vi "Coaxial RF generator control.vi"() -> ()   [LabVIEW 2021]
uses:
  <vilib>/LabVIEW Interface for Arduino/Type Defs/Pin Mode.ctl
  <vilib>/LabVIEW Interface for Arduino/LabVIEW Interface for Arduino.lvlib
panel:
  in  "Generator on/off":bool
  out "Plasma OFF":bool
  out "NOT signal":bool
  out "Plasma ON":bool
  in  "Enable RF On":bool
  in  "Set power / %":dbl min=0.0 max=100.0 step=0.2
  in  "Turn plasma On":bool
  in  "Enable Set Power":bool
  out "Fwd power":dbl format="%#.1g"
  out "Ref power":dbl format="%#.1g"
  out "Ref power":dbl(knob) scale=0.0..15.0
  out "Fwd power":u32(knob) scale=0.0..150.0
  out "error out":errorcluster
  in  "Stopp":bool
  # "Plasma"
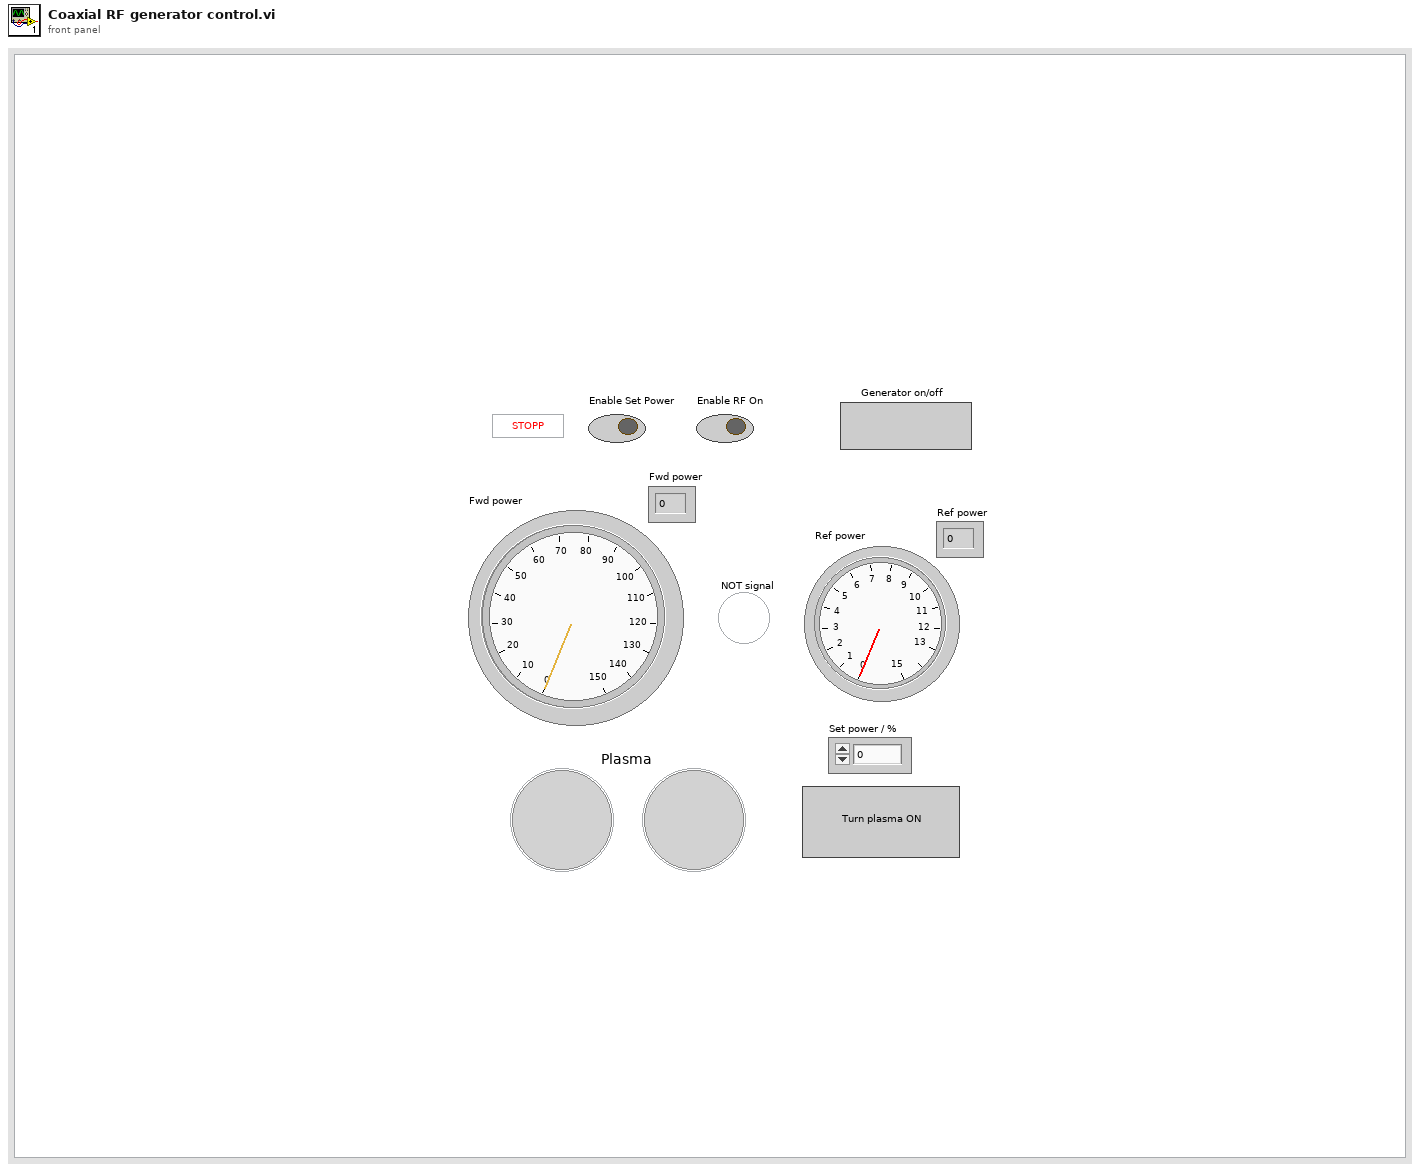
[diagram p1: front panel]
types:
  T1 = typedef "LabVIEW Interface for Arduino.lvlib/Pin Mode.ctl" = enum8{"Input", "Output"}
  T2 = typedef "LabVIEW Interface for Arduino.lvlib/Arduino Resource.ctl" = cluster{"VISA resource":refnum<visa-resource-name>, "Board Type":T3, "Connection Type":enum8{"USB / Serial"}, "Bytes Per Packet (15)":u8}
  T3 = typedef "LabVIEW Interface for Arduino.lvlib/Board Type.ctl" = enum16{"Uno", "Dimuelanove w/Atmega 328", "Mega 2560"}
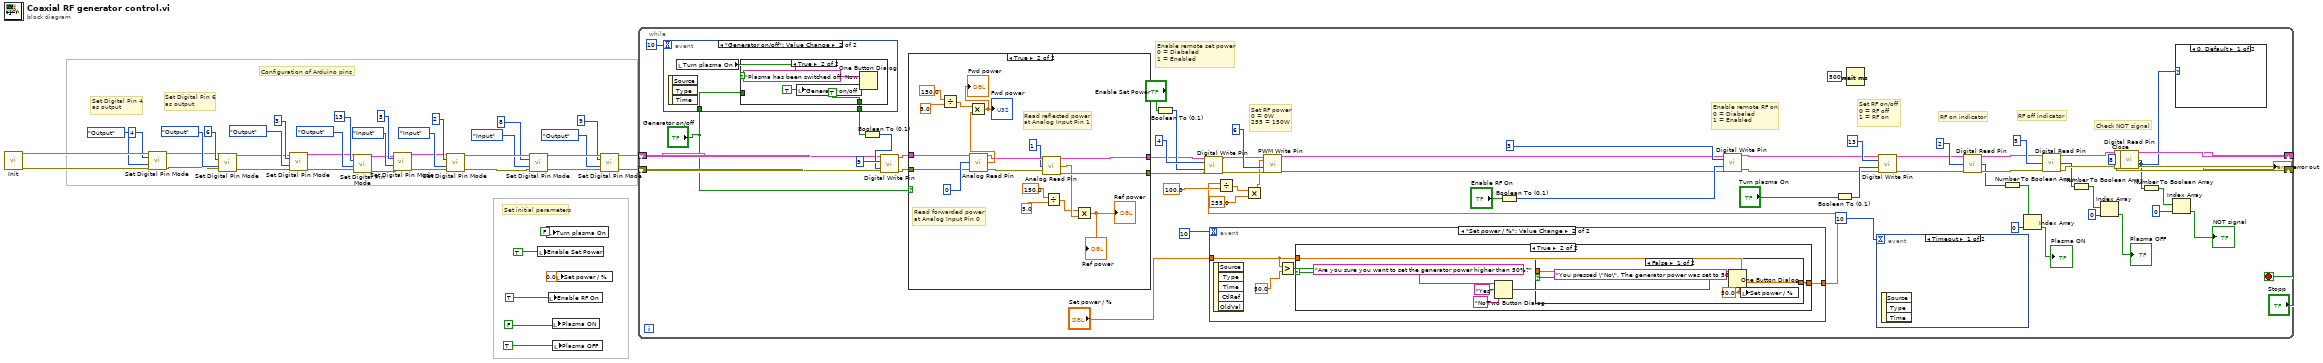
[diagram p0: block diagram]
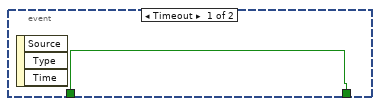
[diagram p2: hidden frame]
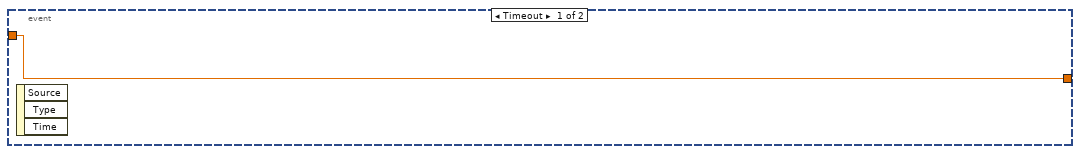
[diagram p4: hidden frame]
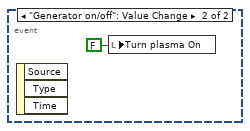
[diagram p8: hidden frame]
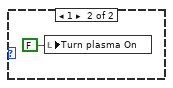
[diagram p9: hidden frame]
diagram:
  # "Configuration of Arduino pins"
  # "Set initial parameters"
  # "Set Digital Pin 6 \nas output"
  # "Set Digital Pin 4 \nas output"
  n1 = call <vilib>:"Init.vi"() -> ("Arduino Resource"=w38:T2, "error out"=w37:errorcluster)  [unwired: 18 in]
  n2 = call <vilib>:"Set Digital Pin Mode.vi"("Arduino Resource"=w38, "Digital I/O Pin"=u8 4, "Pin Mode (Input)"=Pin_Mode."Output", "error in"=w37) -> ("Arduino Resource"=w34:T2, "error out"=w33:errorcluster)  [unwired: 10 in]
  n3 = call <vilib>:"Set Digital Pin Mode.vi"("Arduino Resource"=w34, "Digital I/O Pin"=u8 6, "Pin Mode (Input)"=Pin_Mode."Output", "error in"=w33) -> ("Arduino Resource"=w26:T2, "error out"=w25:errorcluster)  [unwired: 10 in]
  n4 = call <vilib>:"Set Digital Pin Mode.vi"("Arduino Resource"=w26, "Digital I/O Pin"=u8 3, "Pin Mode (Input)"=Pin_Mode."Output", "error in"=w25) -> ("Arduino Resource"=w27:T2, "error out"=w28:errorcluster)  [unwired: 10 in]
  n5 = call <vilib>:"Set Digital Pin Mode.vi"("Arduino Resource"=w27, "Digital I/O Pin"=u8 13, "Pin Mode (Input)"=Pin_Mode."Output", "error in"=w28) -> ("Arduino Resource"=w22:T2, "error out"=w21:errorcluster)  [unwired: 10 in]
  n6 = call <vilib>:"Set Digital Pin Mode.vi"("Arduino Resource"=w22, "Digital I/O Pin"=u8 5, "Pin Mode (Input)"=Pin_Mode."Input", "error in"=w21) -> ("Arduino Resource"=w18:T2, "error out"=w17:errorcluster)  [unwired: 10 in]
  n7 = call <vilib>:"Set Digital Pin Mode.vi"("Arduino Resource"=w18, "Digital I/O Pin"=u8 2, "Pin Mode (Input)"=Pin_Mode."Input", "error in"=w17) -> ("Arduino Resource"=w8:T2, "error out"=w7:errorcluster)  [unwired: 10 in]
  n8 = call <vilib>:"Set Digital Pin Mode.vi"("Arduino Resource"=w8, "Digital I/O Pin"=u8 8, "Pin Mode (Input)"=Pin_Mode."Input", "error in"=w7) -> ("Arduino Resource"=w12:T2, "error out"=w11:errorcluster)  [unwired: 10 in]
  n9 = local write "Enable Set Power"(TRUE ("Enable Set Power")) -> ()
  n10 = local write "Turn plasma On"(FALSE ("Plasma ON")) -> ()
  n11 = local write "Enable RF On"(TRUE ("Enable RF On")) -> ()
  n12 = local write "Plasma ON"(FALSE ("Plasma ON")) -> ()
  n13 = local write "Plasma OFF"(TRUE ("Plasma OFF")) -> ()
  n14 = local write "Set power / %"(0.0 ("Set power")) -> ()
  n15 = call <vilib>:"Set Digital Pin Mode.vi"("Arduino Resource"=w12, "Digital I/O Pin"=u8 9, "Pin Mode (Input)"=Pin_Mode."Output", "error in"=w11) -> ("Arduino Resource"=w10:T2, "error out"=w9:errorcluster)  [unwired: 10 in]
  n16 = while {
    shift-right: [w54] -> w16
    shift-left: w10 -> [w57]
    shift-right: [w55] -> w15
    shift-left: w9 -> [w56]
    stop <- "Stopp" stop-if-true
    # "Check NOT signal"
    # "RF off indicator"
    # "RF on indicator"
    # "Set RF on/off\n0 = RF off\n1 = RF on"
    # "Enable remote RF on \n0 = Diabaled\n1 = Enabled"
    # "Enable remote set power \n0 = Diabaled\n1 = Enabled"
    # "Set RF power\n0 = 0W\n255 = 150W"
    n17 = event shown="[1] \"Generator on/off\": Value Change" {
      selector: _ -> [_ _]
      dyn-events: _ -> [_ _]
      timeout: 10 -> [_ _]
      tunnel: "Generator on/off" -> [w104 w106]
      tunnel: [w104 w105] -> w44
      event Timeout {
        n18 = event-data() -> ()  [unwired: 1 in, 3 out]
      }
      event "Generator on/off": Value Change {
        n19 = event-data() -> ()  [unwired: 1 in, 3 out]
        n20 = local read "Turn plasma On"() -> (w107:bool)
        n21 = case shown="True" w107 {
          tunnel: w106 -> [w108 _]
          tunnel: [w108 TRUE ("Generator on/off")] -> w105
          frame False {
          }
          frame True {
            n22 = local write "Generator on/off"(TRUE ("Generator on/off")) -> ()
            n23 = One Button Dialog(message="Plasma has been switched off. Now the generator can be switched off." ("Nachricht")) -> ()  [unwired: 1 in, 1 out]
          }
        }
      }
    }
    n24 = Boolean To (0,1)(Boolean=w44) -> (0, 1=w60:i16)
    n25 = call <vilib>:"Digital Write Pin.vi"("Arduino Resource"=w57, "Digital I/O Pin (0)"=u8 9, "Value (0)"=w60, "error in"=w56) -> ("Arduino Resource"=w59:T2, "error out"=w58:errorcluster)  [unwired: 10 in]
    n26 = case shown="True" "Generator on/off" {
      tunnel: w59 -> [w128 w140]
      tunnel: w58 -> [w127 w139]
      tunnel: [w128 w136] -> w91
      tunnel: [w127 w135] -> w90
      frame False {
      }
      frame True {
        # "Read reflected power \nat Analog Input Pin 1"
        # "Read forwarded power \nat Analog Input Pin 0"
        n27 = Divide(x=150.0, y=5.0) -> (x/y=w142:dbl)
        n28 = call <vilib>:"Analog Read Pin.vi"("Arduino Resource"=w140, "Analog Input Pin (0)"=u8 0, "error in"=w139) -> ("Arduino Resource"=w138:T2, "Voltage"=w143:dbl, "error out"=w137:errorcluster)  [unwired: 10 in]
        n29 = Multiply(x=w142, y=w143) -> (x*y=→"Fwd power" →"Fwd power":dbl)
        n30 = call <vilib>:"Analog Read Pin.vi"("Arduino Resource"=w138, "Analog Input Pin (0)"=u8 1, "error in"=w137) -> ("Arduino Resource"=w136:T2, "Voltage"=w131:dbl, "error out"=w135:errorcluster)  [unwired: 10 in]
        n31 = Divide(x=150.0, y=5.0) -> (x/y=w130:dbl)
        n32 = Multiply(x=w130, y=w131) -> (x*y=→"Ref power" →"Ref power":dbl)
      }
    }
    n33 = Boolean To (0,1)(Boolean="Enable Set Power") -> (0, 1=w99:i16)
    n34 = call <vilib>:"Digital Write Pin.vi"("Arduino Resource"=w91, "Digital I/O Pin (0)"=u8 4, "Value (0)"=w99, "error in"=w90) -> ("Arduino Resource"=w89:T2, "error out"=w88:errorcluster)  [unwired: 10 in]
    n35 = event shown="[1] \"Set power / %\": Value Change" {
      selector: _ -> [_ _]
      dyn-events: _ -> [_ _]
      timeout: 10 -> [_ _]
      tunnel: "Set power / %" -> [w112 w113]
      tunnel: [w112 w114] -> w49
      event Timeout {
        n36 = event-data() -> ()  [unwired: 1 in, 3 out]
      }
      event "Set power / %": Value Change {
        n37 = event-data() -> ()  [unwired: 1 in, 5 out]
        n38 = Greater?(x=w113, y=50.0) -> (0:w115:bool)
        n39 = case shown="True" w115 {
          tunnel: [w117 w120] -> w114
          tunnel: w113 -> [w117 w121]
          frame False {
          }
          frame True {
            n40 = Two Button Dialog(message="Are you sure you want to set the generator power higher than 50%?" ("Nachricht"), 1:"No" ("Text für F-Schaltfläche (\"Abbrechen\")"), 2:"Yes" ("Text für T-Schaltfläche (\"OK\")")) -> (T button?=w122:bool)
            n41 = case shown="False" w122 {
              tunnel: w121 -> [_ w126]
              tunnel: [w125 w126] -> w120
              frame False {
                w125 = 50.0 ("Set power / %")
                n42 = One Button Dialog(message="You pressed \"No\". The generator power was set to 50%" ("Nachricht")) -> ()  [unwired: 1 in, 1 out]
                n43 = local write "Set power / %"(w125) -> ()
              }
              frame True {
              }
            }
          }
        }
      }
    }
    n44 = Divide(x=w49, y=100.0) -> (x/y=w53:dbl)
    n45 = Multiply(x=w53, y=255.0) -> (x*y=w51:dbl)
    n46 = call <vilib>:"PWM Write Pin.vi"("Arduino Resource"=w89, "Duty Cycle (0 - 255)"=w51, "PWM Pin (3)"=u8 6, "error in"=w88) -> ("Arduino Resource"=w87:T2, "error out"=w86:errorcluster)  [unwired: 10 in]
    n47 = Boolean To (0,1)(Boolean="Enable RF On") -> (0, 1=w93:i16)
    n48 = call <vilib>:"Digital Write Pin.vi"("Arduino Resource"=w87, "Digital I/O Pin (0)"=u8 3, "Value (0)"=w93, "error in"=w86) -> ("Arduino Resource"=w84:T2, "error out"=w85:errorcluster)  [unwired: 10 in]
    n49 = Boolean To (0,1)(Boolean="Turn plasma On") -> (0, 1=w98:i16)
    n50 = Wait (ms)(milliseconds to wait=u32 500 ("Zu wartende ms")) -> ()  [unwired: 1 out]
    n51 = event shown="[0] Timeout" {
      selector: _ -> [_ _]
      dyn-events: _ -> [_ _]
      timeout: 10 -> [_ _]
      event Timeout {
        n52 = event-data() -> ()  [unwired: 1 in, 3 out]
      }
      event "Generator on/off": Value Change {
        n53 = event-data() -> ()  [unwired: 1 in, 3 out]
        n54 = local write "Turn plasma On"(FALSE ("Plasma ON")) -> ()
      }
    }
    n55 = call <vilib>:"Digital Write Pin.vi"("Arduino Resource"=w84, "Digital I/O Pin (0)"=u8 13, "Value (0)"=w98, "error in"=w85) -> ("Arduino Resource"=w79:T2, "error out"=w82:errorcluster)  [unwired: 10 in]
    n56 = call <vilib>:"Digital Read Pin.vi"("Arduino Resource"=w79, "Digital I/O Pin (0)"=u8 2, "error in"=w82) -> ("Arduino Resource"=w80:T2, "Value"=w78:u8, "error out"=w81:errorcluster)  [unwired: 10 in]
    n57 = Number To Boolean Array(number=w78) -> (Boolean array=w73:bool[])
    n58 = Index Array(array=w73, index=0 ("Index")) -> (element=→"Plasma ON":bool)
    n59 = call <vilib>:"Digital Read Pin.vi"("Arduino Resource"=w80, "Digital I/O Pin (0)"=u8 5, "error in"=w81) -> ("Arduino Resource"=w77:T2, "Value"=w70:u8, "error out"=w76:errorcluster)  [unwired: 10 in]
    n60 = Number To Boolean Array(number=w70) -> (Boolean array=w69:bool[])
    n61 = Index Array(array=w69, index=0 ("Index")) -> (element=→"Plasma OFF":bool)
    n62 = call <vilib>:"Digital Read Pin.vi"("Arduino Resource"=w77, "Digital I/O Pin (0)"=u8 8, "error in"=w76) -> ("Arduino Resource"=w54:T2, "Value"=w74:u8, "error out"=w55:errorcluster)  [unwired: 10 in]
    n63 = Number To Boolean Array(number=w74) -> (Boolean array=w65:bool[])
    n64 = Index Array(array=w65, index=0 ("Index")) -> (element=→"NOT signal":bool)
    n65 = case shown="0, Default" w74 {
      frame 0, Default {
      }
      frame 1 {
        n66 = local write "Turn plasma On"(FALSE ("Plasma ON")) -> ()
      }
    }
  }
  n67 = call <vilib>:"Close.vi"("Arduino Resource"=w16, "error in"=w15) -> ("error out"=→"error out":errorcluster)  [unwired: 13 in]
